vi "CheckError.vi"(1 "error in (no error)":errorcluster, 2 "ret_val":bool) -> (0 "error out":errorcluster)   [LabVIEW 2015]
uses:
  XGL_DPP.lvlib
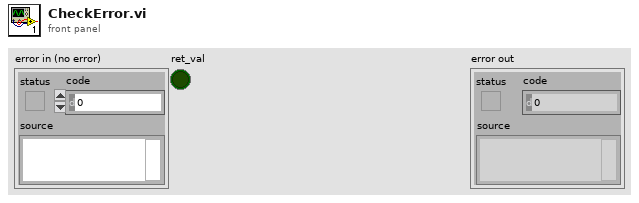
[diagram p1: front panel]
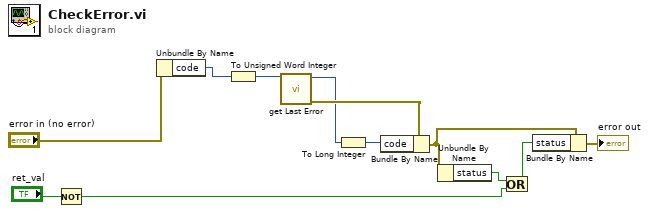
[diagram p0: block diagram]
diagram:
  n1 = Not(x="ret_val") -> (.not. x?=w4:bool)
  n2 = Unbundle By Name("error in (no error)") -> ("code"=w12:i32)
  n3 = To Unsigned Word Integer(number=w12) -> (unsigned 16bit integer=w11:u16)
  n4 = call "get Last Error.vi"("error_code"=w11) -> ("error out"=w10:errorcluster, "error_code out"=w8:u16)  [unwired: 8 in, 1 out]
  n5 = To Long Integer(number=w8) -> (32bit integer=w9:i32)
  n6 = Bundle By Name(cluster=w10, "code"=w9) -> (w2:errorcluster)
  n7 = Unbundle By Name(w2) -> ("status"=w5:bool)
  n8 = Or(x=w5, y=w4) -> (x .or. y?=w3:bool)
  n9 = Bundle By Name(cluster=w2, "status"=w3) -> (→"error out":errorcluster)
